vi "KBActive.vi"(0 "device ID":refnum<k1>, 1 "M3 decreasing":i32, 2 "M3 increasing":i32, 3 "M1 increasing":i32, 4 "M1 decreasing":i32, 5 "M2 decreasing":i32, 6 "M2 increasing":i32) -> ()   [LabVIEW 2020]
uses:
  <vilib>/Utility/inputDevices.llb/keyboardAcquire.vi
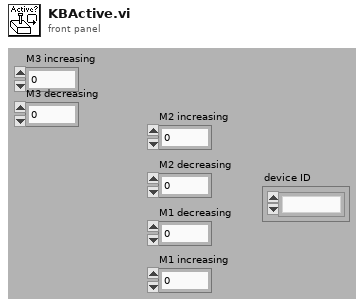
[diagram p1: front panel]
types:
  T1 = enum16{"0", "1", "2", "3", "4", "5", "6", "7", "8", "9", "A", "B", "C", "D", "E", "F", "G", "H", "I", "J", "K", "L", "M", "N", "O", "P", "Q", "R", "S", "T", "U", "V", "W", "X", "Y", "Z", "F1", "F2", "F3", "F4", "F5", "F6", "F7", "F8", "F9", "F10", "F11", "F12", "F13", "F14", "F15", "ADD", "BACK", "BACKSLASH", "CAPITAL", "COMMA", "DECIMAL", "DELETE", "DIVIDE", "DOWN", "END", "EQUALS", "ESCAPE", "GRAVE (`)", "HOME", "INSERT", "LBRACKET", "LCONTROL", "LEFT", "L ALT", "LSHIFT", "LWIN", "MINUS", "MULTIPLY", "NEXT", "NUMLOCK", "NUMPAD_0", "NUMPAD_1", "NUMPAD_2", "NUMPAD_3", "NUMPAD_4", "NUMPAD_5", "NUMPAD_6", "NUMPAD_7", "NUMPAD_8", "NUMPAD_9", "PAUSE", "PERIOD", "PRIOR (PG UP)", "RBRACKET", "RCONTROL", "RETURN", "RIGHT", "R ALT", "RSHIFT", "RWIN", "SCROLL", "SEMICOLON", "SLASH", "SPACE", "SUBTRACT", "TAB", "UP", "ENTER (num pad)", "' (quote)"}[]
  T2 = enum16{"0", "1", "2", "3", "4", "5", "6", "7", "8", "9", "A", "B", "C", "D", "E", "F", "G", "H", "I", "J", "K", "L", "M", "N", "O", "P", "Q", "R", "S", "T", "U", "V", "W", "X", "Y", "Z", "F1", "F2", "F3", "F4", "F5", "F6", "F7", "F8", "F9", "F10", "F11", "F12", "F13", "F14", "F15", "ADD", "BACK", "BACKSLASH", "CAPITAL", "COMMA", "DECIMAL", "DELETE", "DIVIDE", "DOWN", "END", "EQUALS", "ESCAPE", "GRAVE (`)", "HOME", "INSERT", "LBRACKET", "LCONTROL", "LEFT", "L ALT", "LSHIFT", "LWIN", "MINUS", "MULTIPLY", "NEXT", "NUMLOCK", "NUMPAD_0", "NUMPAD_1", "NUMPAD_2", "NUMPAD_3", "NUMPAD_4", "NUMPAD_5", "NUMPAD_6", "NUMPAD_7", "NUMPAD_8", "NUMPAD_9", "PAUSE", "PERIOD", "PRIOR (PG UP)", "RBRACKET", "RCONTROL", "RETURN", "RIGHT", "R ALT", "RSHIFT", "RWIN", "SCROLL", "SEMICOLON", "SLASH", "SPACE", "SUBTRACT", "TAB", "UP", "ENTER (num pad)", "' (quote)"}
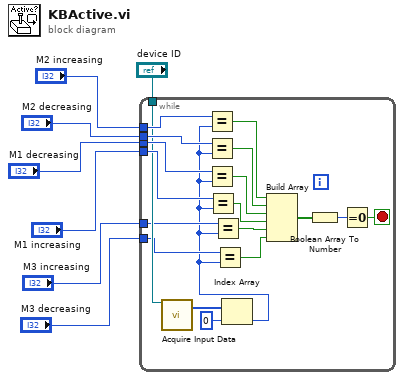
[diagram p0: block diagram]
diagram:
  n1 = while {
    tunnel: "device ID" -> [w13]
    tunnel: "M1 increasing" -> [w17]
    tunnel: "M1 decreasing" -> [w16]
    tunnel: "M2 decreasing" -> [w15]
    tunnel: "M2 increasing" -> [w14]
    tunnel: "M3 increasing" -> [w12]
    tunnel: "M3 decreasing" -> [w10]
    stop <- w19 stop-if-true
    n2 = call-poly <vilib>:"Acquire Input Data.vi"("device ID"=w13) -> ("keys pressed"=w25:T1)  [unwired: 1 in, 17 out]
    n3 = Index Array(array=w25, index=0) -> (element=w9:T2)
    n4 = Equal?(x=w14, y=w9) -> (x = y?=w21:bool)
    n5 = Equal?(x=w15, y=w9) -> (x = y?=w22:bool)
    n6 = Equal?(x=w16, y=w9) -> (x = y?=w23:bool)
    n7 = Equal?(x=w17, y=w9) -> (x = y?=w24:bool)
    n8 = Equal?(x=w12, y=w9) -> (x = y?=w11:bool)
    n9 = Equal?(x=w10, y=w9) -> (x = y?=w8:bool)
    n10 = Build Array(w21, w22, w23, w24, w11, w8) -> (w20:bool[])
    n11 = Boolean Array To Number(Boolean array=w20) -> (number=w18:u32)
    n12 = Equal To 0?(x=w18) -> (x = 0?=w19:bool)
  }
